vi "Byte Array to Hex String.vi"(1 "bytes array":u8[](array[numeric])) -> (0 "hex string":string)   [LabVIEW 2013]
doc: "Converts <b>bytes array</b> into <b>hex string</b> (seen as a hexadecimal string in \"normal display\")."
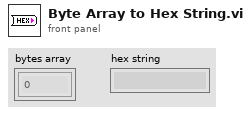
[diagram p1: front panel]
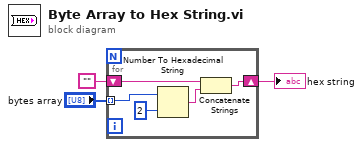
[diagram p0: block diagram]
diagram:
  n1 = for {
    tunnel: "bytes array" -> [w8] mode=indexing
    shift-right: [w5] -> w3
    shift-left: "" -> [w4]
    n2 = Number To Hexadecimal String(1:i16 2 ("width (-)"), 2:w8) -> (0:w6:string)
    n3 = Concatenate Strings(w4, w6) -> (w5:string)
  }
  "hex string" <- w3
